vi "Write General Settings.vi"(8 "error in":errorcluster, 10 "General":T1) -> (0 "error out":errorcluster)   [LabVIEW 2011, in "GraphicalTestRunner.lvlib"]
uses:
  GraphicalTestRunner.lvlib
  <vilib>/Utility/config.llb/NI_LVConfig.lvlib
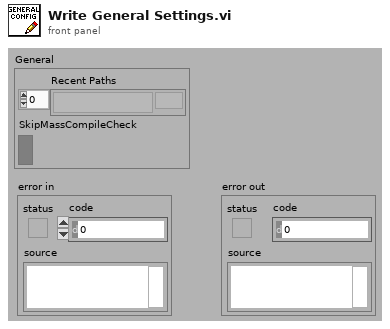
[diagram p1: front panel]
types:
  T1 = cluster{"Recent Paths":path[], "SkipMassCompileCheck":bool}
  T2 = typedef "NI_LVConfig.lvlib/Config Data RefNum.ctl" = refnum<k1>
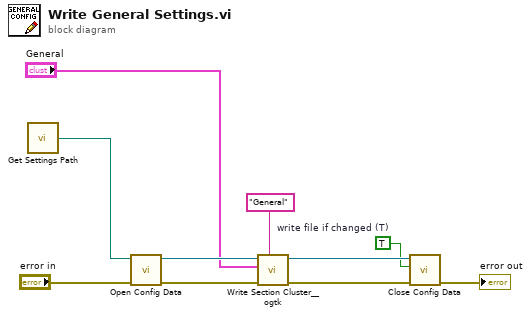
[diagram p0: block diagram]
diagram:
  w2 = TRUE  # write file if changed (T)
  n1 = call "Get Settings Path.vi"() -> ("config path"=w4:path)
  n2 = call <vilib>:"Open Config Data.vi"("error in (no error)"="error in", "configuration file path"=w4) -> ("error out"=w9:errorcluster, "refnum"=w6:T2)  [unwired: 7 in, 1 out]
  n3 = call <userlib>:"Write Section Cluster__ogtk.vi"("section (optional)"="General", "error in (no error)"=w9, "Section Formatted Cluster"="General", "refnum"=w6) -> ("error out"=w8:errorcluster, "dup refnum"=w5:T2)  [unwired: 6 in]
  n4 = call <vilib>:"Close Config Data.vi"("error in (no error)"=w8, "write file if changed (T)"=w2, "refnum"=w5) -> ("error out"=→"error out":errorcluster)  [unwired: 7 in, 1 out]
